vi "数据采集1channel默认保存路径更改.vi"() -> ()   [LabVIEW 2018]
uses:
  <vilib>/Waveform/WDTOps.llb/WDT Get Waveform Time Array DBL.vi
  <vilib>/Utility/file.llb/Write Delimited Spreadsheet (DBL).vi
panel:
  out "波形图 4":dynamicdata(graph)
  out "波形图 3":dynamicdata(graph)
  out "波形图 2":dynamicdata(graph)
  in  "文件路径（使用对话框）":path=path "C:/Users/86136/source/repos/Vt of temp.txt"
  out "error out":errorcluster caption="错误输出"
  out "Voltage":cluster{"Y":dbl[], "Y":dbl[]}[](graph)
  out "波形图":dynamicdata(graph)
  out "波形图表":dynamicdata(graph)
  in  "File Name":string
  in  "File Path":path
  in  "stop (F)":bool caption="停止(F)"
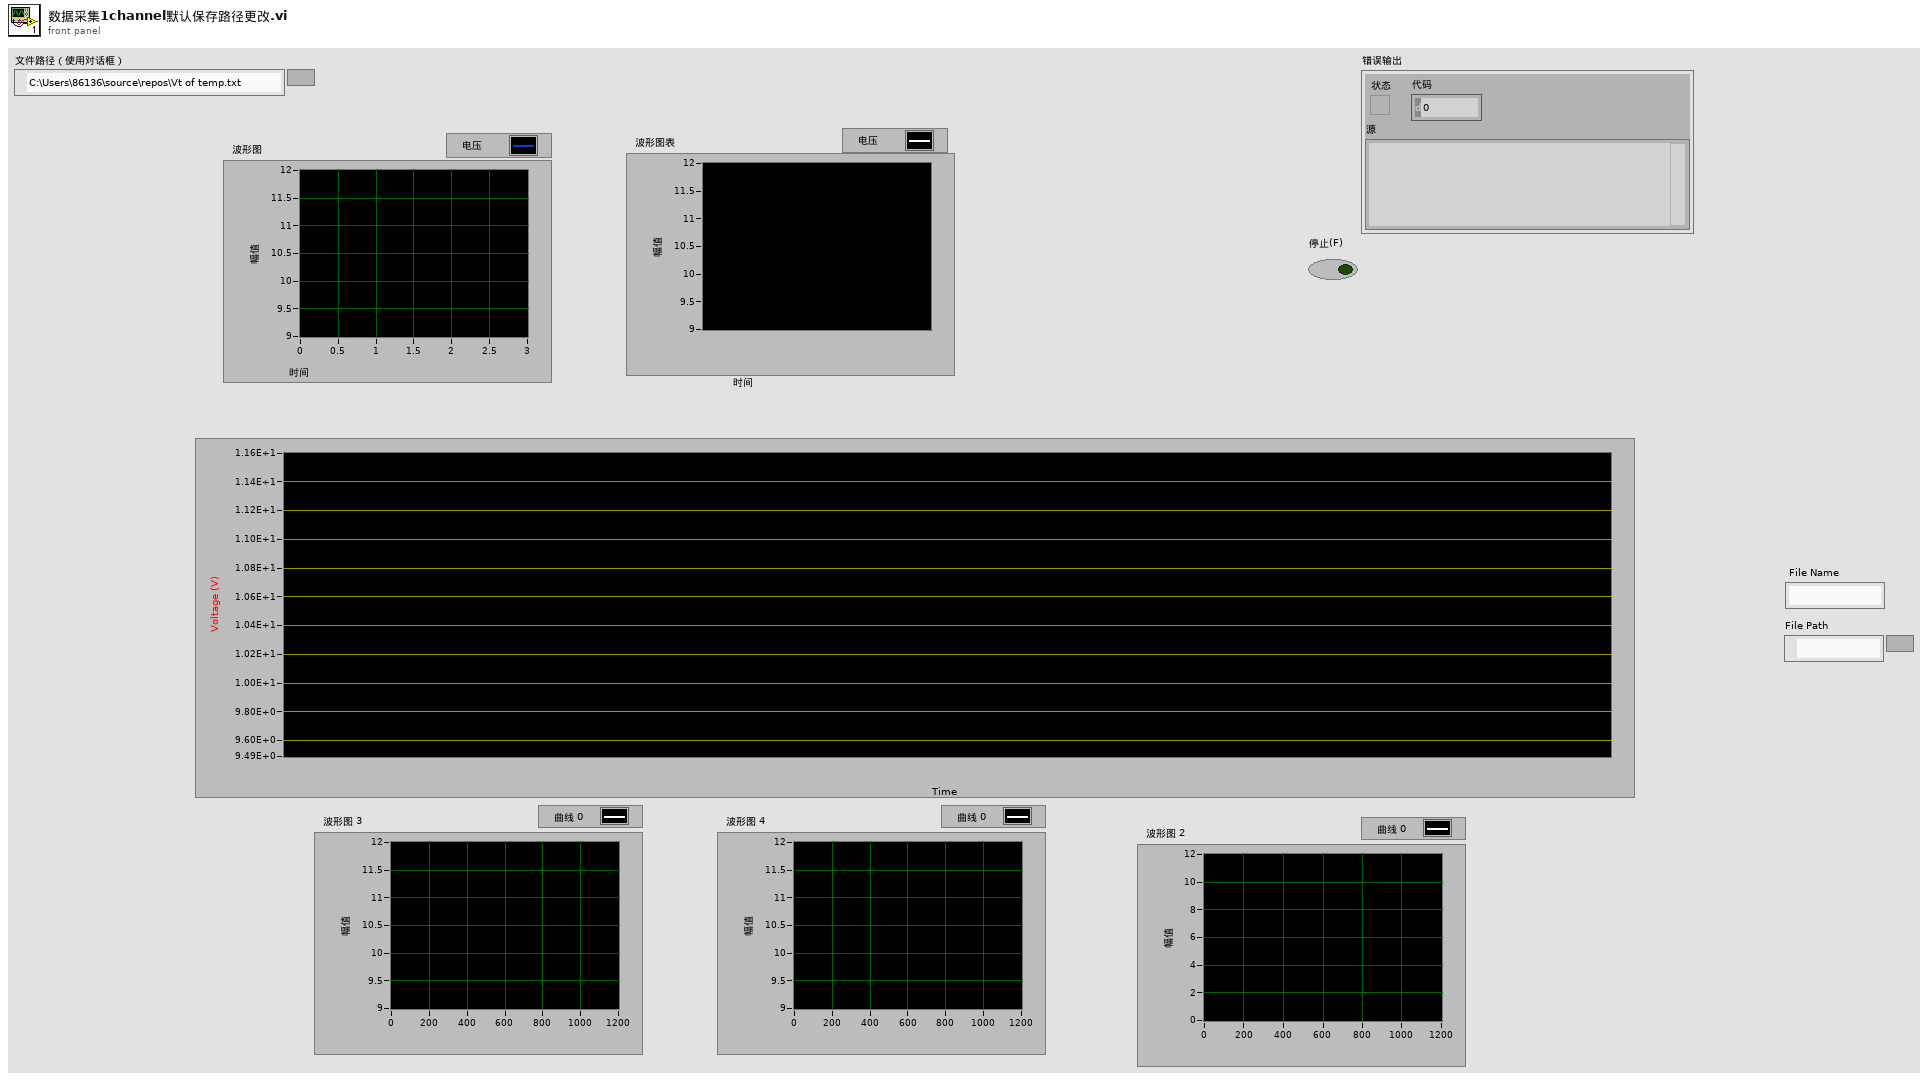
[diagram p1: front panel]
types:
  T1 = enum16{"open", "replace", "create", "open or create", "replace or create", "replace or create with confirmation"}
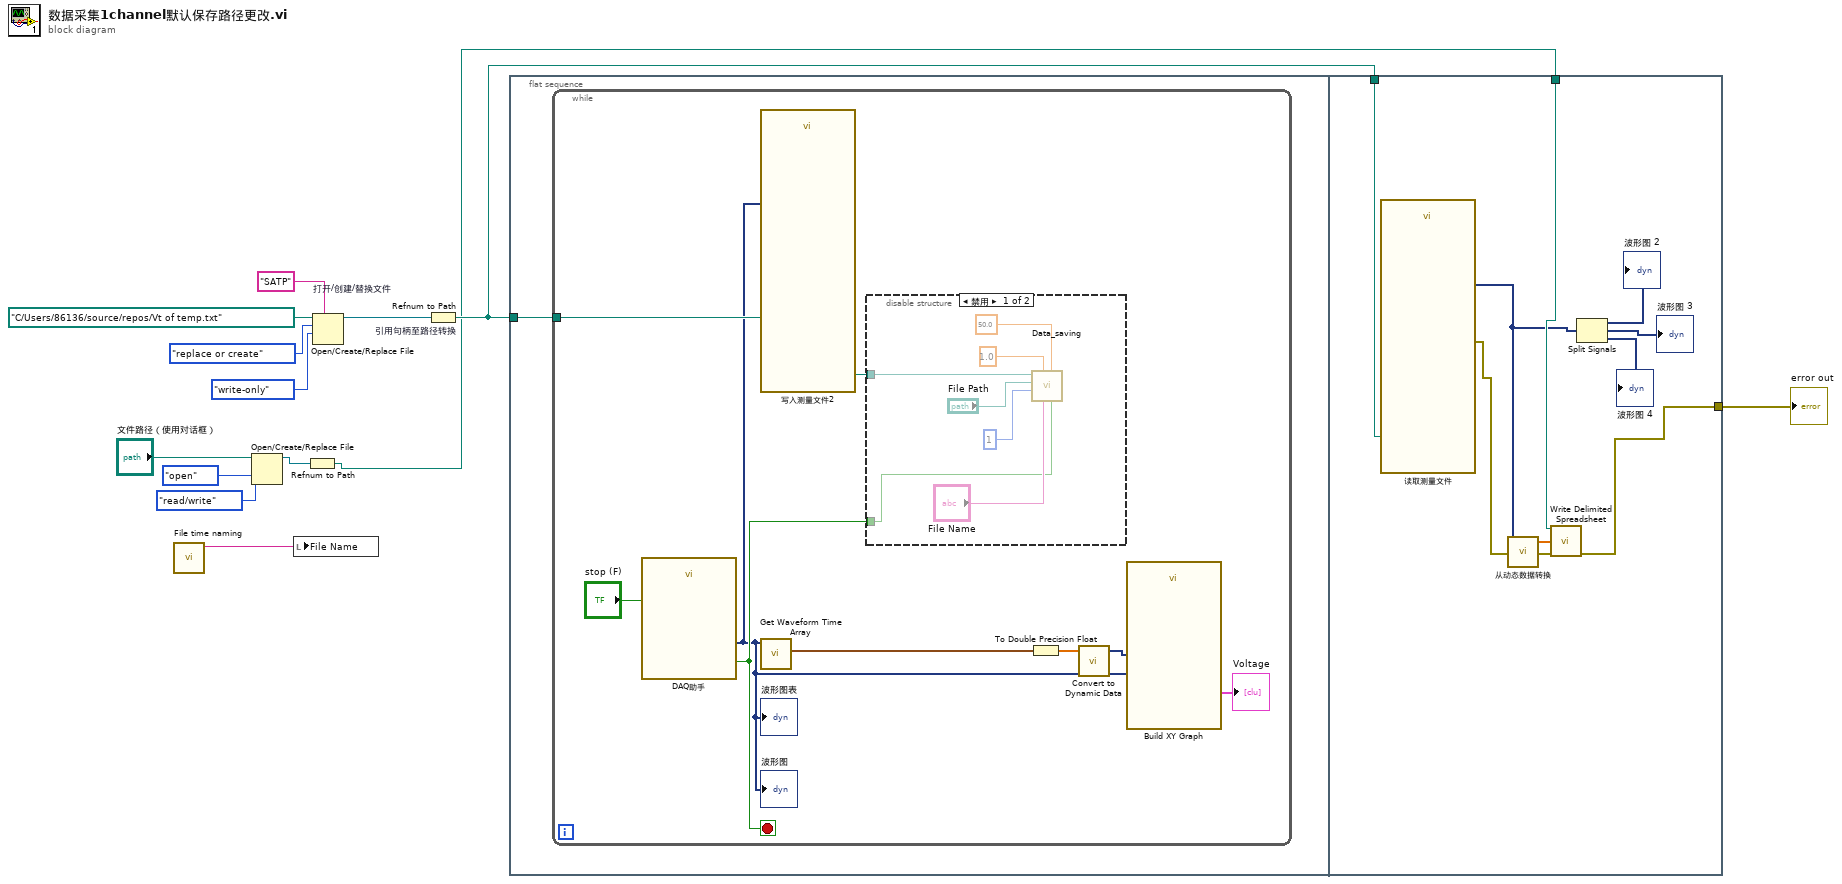
[diagram p0: block diagram]
diagram:
  n1 = call "File time naming.vi"() -> ("result string"=w13:string)  [unwired: 11 in]
  n2 = Open/Create/Replace File(file path (use dialog)="文件路径（使用对话框）", operation (0:open)=T1."open" ("操作(0:open)"), access (0:read/write)=enum16{"read/write", "read-only", "write-only"}."read/write" ("权限(0:read/write)")) -> (refnum out=w2:refnum<file>)  [unwired: 3 in, 2 out]
  n3 = local write "File Name"(w13) -> ()
  n4 = Refnum to Path(1:w2) -> (0:w1:path)
  n5 = Open/Create/Replace File "打开/创建/替换文件"(file path (use dialog)=path "C:/Users/86136/source/repos/Vt of temp.txt" ("文件路径（使用对话框）"), prompt="SATP" ("提示"), operation (0:open)=T1."replace or create" ("操作(0:open)"), access (0:read/write)=enum16{"read/write", "read-only", "write-only"}."write-only" ("权限(0:read/write)")) -> (refnum out=w9:refnum<file>)  [unwired: 2 in, 2 out]
  n6 = Refnum to Path "引用句柄至路径转换"(1:w9) -> (0:w7:path)
  n7 = flat-sequence {
    tunnel: w7 -> [w14]
    tunnel: w7 -> [w39]
    tunnel: w1 -> [w38]
    tunnel: [w35] -> w6
    frame #0 {
      n8 = while {
        tunnel: w14 -> [w22]
        stop <- w20 stop-if-true
        n9 = call "DAQ助手"("stop (F)"="stop (F)") -> ("data"=w15:dynamicdata, "stopped"=w20:bool)  [unwired: 15 in, 2 out]
        "波形图表" <- w15
        "波形图" <- w15
        n10 = call "写入测量文件2"("Signals"=w15, "Filename"=w22) -> ("Filename Out"=w23:path)  [unwired: 15 in, 2 out]
        n11 = call-poly <vilib>:"Get Waveform Time Array.vi"("waveform in"=w15) -> ("X array"=w19:timestamp[])  [unwired: 1 in, 9 out]
        n12 = disable-structure shown="禁用" {
          disable-tunnel: w23 -> [w25 _]
          disable-tunnel: w20 -> [w24 _]
          frame Disabled {
            n13 = call "Data_saving.vi"("Boolean"=w24, "Sampling Rate"=50.0, "File Name"="File Name", "Voltage Sensitivity\n1000 will be 1000"=1.0 ("Voltage Sensitivity\n1000 will be 1000"), "Number of Samples Per Channel"=1, "File Path"="File Path", "File name source"=w25) -> ()  [unwired: 5 in]
          }
          frame Enabled {
          }
        }
        n14 = To Double Precision Float(number=w19) -> (double precision float=w18:dbl[])
        n15 = call "Convert to Dynamic Data"("Array"=w18) -> ("Dynamic Data Type"=w17:dynamicdata)  [unwired: 3 out]
        n16 = call "Build XY Graph"("Y Input"=w15, "X Input"=w17) -> ("XY Graph"=→"Voltage":cluster{"Y":dbl[], "Y":dbl[]}[])  [unwired: 3 in, 6 out]
      }
    }
    frame #1 {
      n17 = call "读取测量文件"("Filename"=w39) -> ("error out"=w36:errorcluster, "Signals"=w34:dynamicdata)  [unwired: 5 in, 4 out]
      n18 = call "从动态数据转换"("Dynamic Data Type"=w34) -> ("Array"=w37:dbl[])  [unwired: 3 in]
      n19 = call-poly <vilib>:"Write Delimited Spreadsheet.vi"("file path (dialog if empty)"=w38, "1D data"=w37, "error in (no error)"=w36) -> ("error out"=w35:errorcluster)  [unwired: 11 in, 1 out]
      n20 = Split Signals(w34) -> (→"波形图 2":dynamicdata, →"波形图 3":dynamicdata, →"波形图 4":dynamicdata)  [unwired: 3 in]
    }
  }
  "error out" <- w6
